vi "Change Column Name.vi"(6 "New Column name":string, 8 "error in (no error)":errorcluster, 9 "selected column path":string, 10 "selected table path":string, 11 "Data.PGSQL in":refnum<class "LV-Data.PGSQL.lvclass">) -> (0 "error out":errorcluster, 3 "Data.PGSQL out":refnum<class "LV-Data.PGSQL.lvclass">)   [LabVIEW 2019, in "LV-Data.PGSQL.lvclass"]
uses:
  LV-Data.PGSQL.lvclass
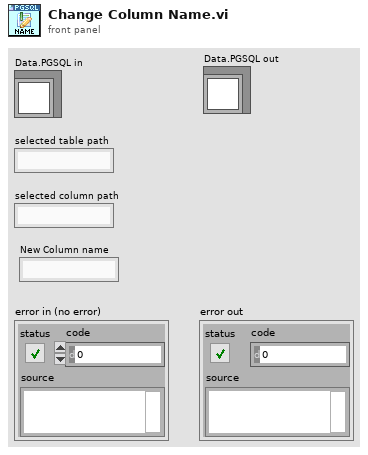
[diagram p1: front panel]
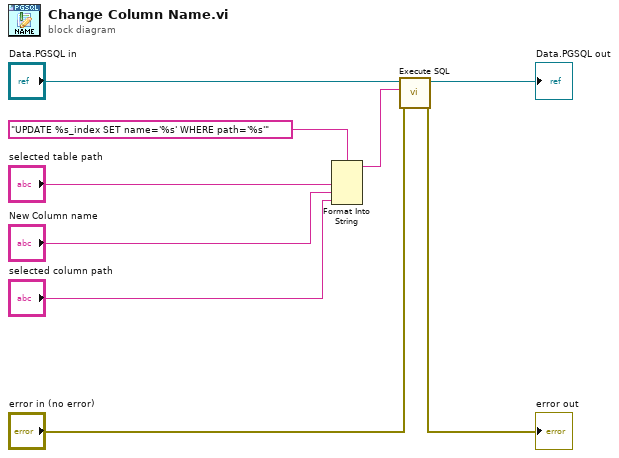
[diagram p0: block diagram]
diagram:
  n1 = Format Into String(format string="UPDATE %s_index SET name='%s' WHERE path='%s'", "selected table path", "New Column name", "selected column path") -> (resulting string=w1:string)  [unwired: 2 in, 1 out]
  n2 = call "Execute SQL.vi"("error in"="error in (no error)", "SQL"=w1, "LV-Data.PGSQL"="Data.PGSQL in") -> ("error out"=→"error out":errorcluster, "LV-Data.PGSQL out"=→"Data.PGSQL out":refnum<class "LV-Data.PGSQL.lvclass">)  [unwired: 5 in, 2 out]
